vi "CRYReport Pic Get CloneVI Name.vi"(11 "sTitle":string) -> (3 "sVIName_Out":string)   [LabVIEW 2013]
uses:
  Kernel32.DLL
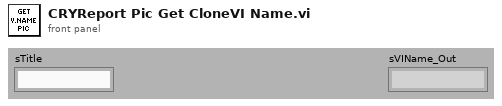
[diagram p1: front panel]
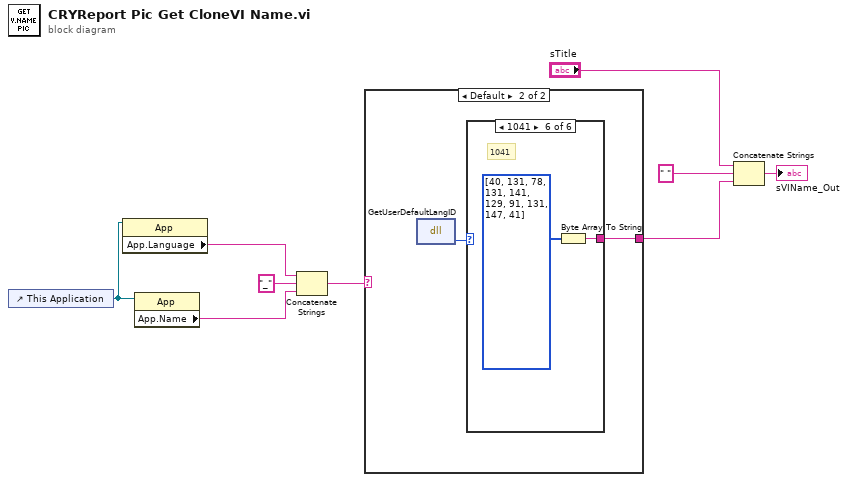
[diagram p0: block diagram]
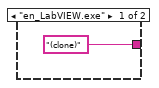
[diagram p2: hidden frame]
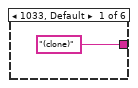
[diagram p3: hidden frame]
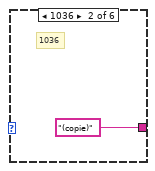
[diagram p4: hidden frame]
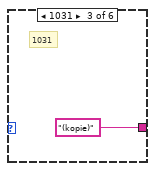
[diagram p5: hidden frame]
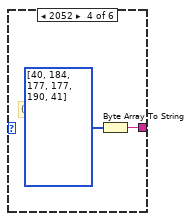
[diagram p6: hidden frame]
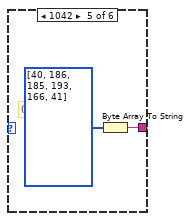
[diagram p7: hidden frame]
diagram:
  n1 = control-ref of="This Application"() -> (w5:refnum<vi>)
  n2 = property class="App"(reference=w5) -> ("App.Language"=w4:string)  [unwired: 1 in, 2 out]
  n3 = property class="App"(reference=w5) -> ("App.Name"=w3:string)  [unwired: 1 in, 2 out]
  n4 = Concatenate Strings(w4, "_" ("string"), w3) -> (w1:string)
  n5 = case shown="Default" w1 {
    tunnel: ["(clone)" ("string") w11] -> w8
    frame "en_LabVIEW.exe" {
    }
    frame Default {
      n6 = dll-call lib="kernel32.dll" fn="GetUserDefaultLangID"() -> ("return type"=w12:i32)  [unwired: 3 in, 2 out]
      n7 = case shown="1041" w12 {
        tunnel: ["(clone)" ("string") "(copie)" ("string") "(kopie)" ("string") w16 w18 w20] -> w11
        frame 1033, Default {
        }
        frame 1036 {
          # "1036"
        }
        frame 1031 {
          # "1031"
        }
        frame 2052 {
          # "(oR,g)"
          n8 = Byte Array To String(unsigned byte array=i32[] [40, 184, 177, 177, 190, 41]) -> (string=w16:string)
        }
        frame 1042 {
          # "(oR,g)"
          n9 = Byte Array To String(unsigned byte array=i32[] [40, 186, 185, 193, 166, 41]) -> (string=w18:string)
        }
        frame 1041 {
          # "1041"
          n10 = Byte Array To String(unsigned byte array=i32[] [40, 131, 78, 131, 141, 129, 91, 131, 147, 41]) -> (string=w20:string)
        }
      }
    }
  }
  n11 = Concatenate Strings("sTitle", " " ("string"), w8) -> (→"sVIName_Out":string)
